vi "Voorbeeld_Grafieken_XY_graph_Waveform_Graph.vi"() -> ()   [LabVIEW 2019]
panel:
  out "Waveform Graph":i32[](graph)
  out "XY Graph":cluster{i32[], i32[]}(graph)
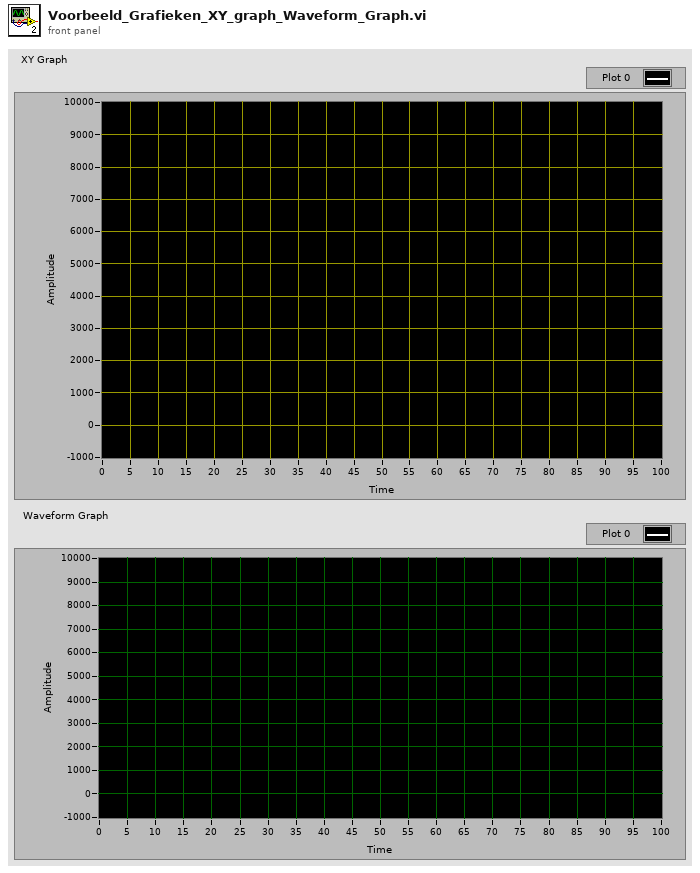
[diagram p1: front panel]
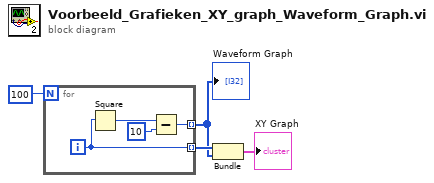
[diagram p0: block diagram]
diagram:
  n1 = for {
    N: 100 -> [_]
    tunnel: [w8] -> w3 mode=indexing
    tunnel: [w5] -> w1 mode=indexing
    i -> [w8]
    n2 = Square(x=w8) -> (x^2=w7:i32)
    n3 = Subtract(x=w7, y=10) -> (x-y=w5:i32)
  }
  "Waveform Graph" <- w1
  n4 = Bundle(w3, w1) -> (→"XY Graph":cluster{i32[], i32[]})  [unwired: 1 in]
